vi "RaF Pre-Import Action.vi"(8 "error in":errorcluster, 10 "sysdef in":T1 {"Tree"."Properties"."Type" items=["K_STRING", "K_BOOL", "K_I32", "K_U32", "K_DOUBLE", "K_U64", "K_VARIANT", "K_DEPENDENTFILE", "K_DEPENDENTNODE", "K_DATASOURCENODE", "K_U16", "K_DBLARR", "K_U32ARR", "K_I32ARR", "K_STRINGARR", "K_DICTIONARY", "K_DICTIONARYARR"]}, 11 "routing and faulting in":T9 format="%.0x") -> (0 "error out":errorcluster, 2 "sysdef out":T1 {"Tree"."Properties"."Type" items=["K_STRING", "K_BOOL", "K_I32", "K_U32", "K_DOUBLE", "K_U64", "K_VARIANT", "K_DEPENDENTFILE", "K_DEPENDENTNODE", "K_DATASOURCENODE", "K_U16", "K_DBLARR", "K_U32ARR", "K_I32ARR", "K_STRINGARR", "K_DICTIONARY", "K_DICTIONARYARR"]}, 3 "routing and faulting out":T9 format="%.0x")   [LabVIEW 2020, in "Routing and Faulting Scripting.lvlib"]
uses:
  Routing and Faulting Scripting.lvlib
  <vilib>/NI VeriStand/Custom Device API/Custom Device Item Ref.ctl
  <vilib>/NI/NI VeriStand Advanced SysDef API/_Types/SysDef.Export.ctl
  <vilib>/NI/NI VeriStand Advanced SysDef API/_Types/TreeItem.ctl
  <vilib>/NI/NI VeriStand Advanced SysDef API/_Types/TreeItem.Info.ctl
  <vilib>/NI VeriStand/Custom Device API/Custom Device Channel.ctl
  <vilib>/NI VeriStand/Custom Device API/Custom Device Channel Type.ctl
  <vilib>/NI VeriStand/Custom Device API/Custom Device Waveform.ctl
  <vilib>/NI VeriStand/Custom Device API/Custom Device Waveform DataType.ctl
  <vilib>/NI/NI VeriStand Advanced SysDef API/_Types/TreeItem.Property.ctl
  <vilib>/NI VeriStand/Custom Device API/Custom Device API.lvlib
  <vilib>/NI/NI VeriStand Advanced SysDef API/SysDef API/Advanced System Definition.lvlib
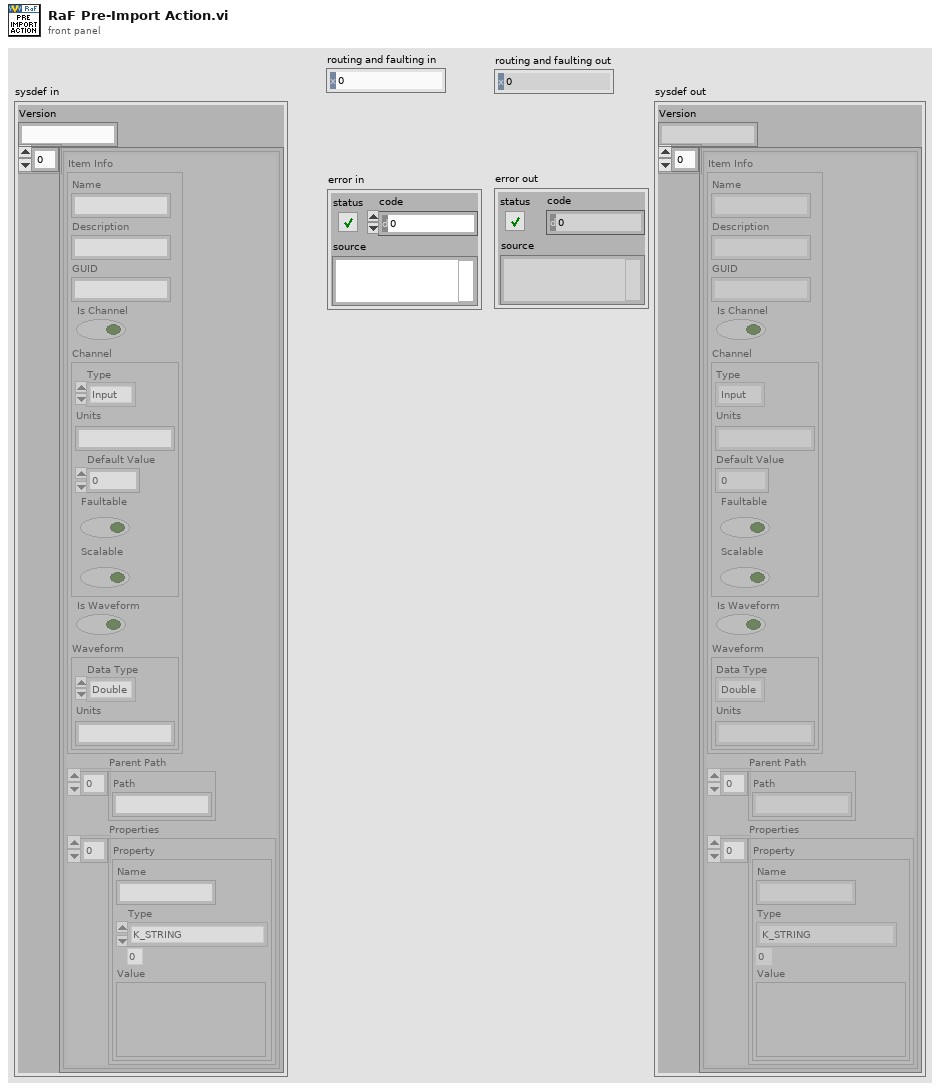
[diagram p1: front panel]
types:
  T1 = typedef "Advanced System Definition.lvlib/SysDef.Export.ctl" = cluster{"Version":string, "Tree":T2[]}
  T2 = typedef "Advanced System Definition.lvlib/TreeItem.ctl" = cluster{"Item Info":T3, "Parent Path":string[], "Properties":T8[]}
  T3 = typedef "Advanced System Definition.lvlib/TreeItem.Info.ctl" = cluster{"Name":string, "Description":string, "GUID":string, "Is Channel":bool, "Channel":T4, "Is Waveform":bool, "Waveform":T6}
  T4 = typedef "Custom Device API.lvlib/Custom Device Channel.ctl" = cluster{"Type":T5, "Units":string, "Default Value":dbl, "Faultable":bool, "Scalable":bool}
  T5 = typedef "Custom Device API.lvlib/Custom Device Channel Type.ctl" = enum16{"Input", "Output"}
  T6 = typedef "Custom Device API.lvlib/Custom Device Waveform.ctl" = cluster{"Data Type":T7, "Units":string}
  T7 = typedef "Custom Device API.lvlib/Custom Device Waveform DataType.ctl" = enum16{"Double", "Complex Double"}
  T8 = typedef "Advanced System Definition.lvlib/TreeItem.Property.ctl" = cluster{"Name":string, "Type":i32, "Value":variant}
  T9 = typedef "Custom Device API.lvlib/Custom Device Item Ref.ctl" = u64
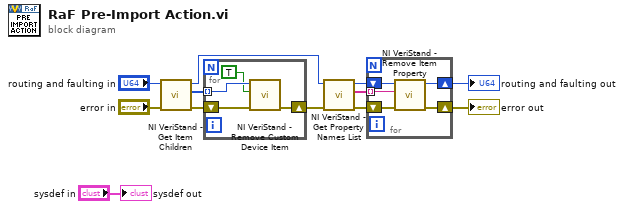
[diagram p0: block diagram]
diagram:
  n1 = call <vilib>:"NI VeriStand - Get Item Children.vi"("error in (no error)"="error in", "Item Ref in"="routing and faulting in") -> ("error out"=w6:errorcluster, "Child Refs"=w7:T9[], "Item Ref out"=w8:T9)  [unwired: 6 in, 1 out]
  n2 = for {
    tunnel: w7 -> [w16] mode=indexing
    shift-right: [w14] -> w5
    shift-left: w6 -> [w15]
    n3 = call <vilib>:"NI VeriStand - Remove Custom Device Item.vi"("error in (no error)"=w15, "Force Delete (F)"=TRUE, "Item Ref in"=w16) -> ("error out"=w14:errorcluster)  [unwired: 7 in, 1 out]
  }
  n4 = call <vilib>:"NI VeriStand - Get Property Names List.vi"("error in (no error)"=w5, "Item Ref in"=w8) -> ("error out"=w9:errorcluster, "Property Names"=w10:string[], "Item Ref out"=w11:T9)  [unwired: 7 in]
  n5 = for {
    tunnel: w10 -> [w20] mode=indexing
    shift-right: [w18] -> w2
    shift-left: w9 -> [w19]
    shift-right: [w17] -> w1
    shift-left: w11 -> [w21]
    n6 = call <vilib>:"NI VeriStand - Remove Item Property.vi"("error in (no error)"=w19, "Property Name"=w20, "Item Ref in"=w21) -> ("error out"=w18:errorcluster, "Item Ref out"=w17:T9)  [unwired: 6 in, 1 out]
  }
  "routing and faulting out" <- w1
  "error out" <- w2
  "sysdef out" <- "sysdef in"
